vi "PH_Switch.destructor.vi"(0 "i ref in":refnum<vi>, 5 "error in(no error)":errorcluster) -> (19 "error out":errorcluster)   [LabVIEW 2014, in "PH_Switch.lvlib"]
doc: "This is the destructor of a class.\n\nLicense Agreement for this software:\n\nCopyright (C)\nGesellschaft für Schwerionenforschung, GSI\nPlanckstr. 1\n64291 Darmstadt\nGermany\n\nContact: D.Beck@gsi.de \n\nThis program is free software; you can redistribute it and/or modify it under the terms of the \nGNU General Public License as published by the Free Software Foundation; either version 2 of \nthe license, or (at your option) any later version.\n\nThis program is distributed in the hope that it will be useful, but WITHOUT ANY WARRANTY; \nwithout even the implied warranty of MERCHANTABILITY or FITNESS FOR A PARTICULAR PURPOSE. See the GNU General License for more details (http://www.gnu.org).\n\nGesellschaft für Schwerionenforschung, GSI\nPlanckstr. 1, 64291 Darmstadt, Germany\nFor all questions and ideas contact: M.Richter@gsi.de, H.Brand@gsi.de or D.Beck@gsi.de.\nLast update: 16-JUN-2004"
uses:
  PH_Switch.lvlib
  PH_PSDBWriter/PH_PSDBWriter.lvlib
  PH_StatusHandler/PH_StatusHandler.lvlib
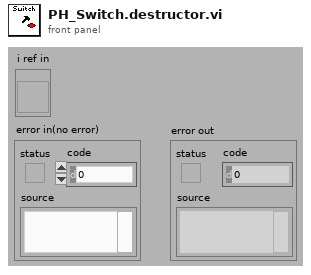
[diagram p1: front panel]
types:
  T1 = enum16{"SetAttribute", "GetAttribute", "CreateAttribute", "DestroyAttribute", "DestroyAllAtributes"}
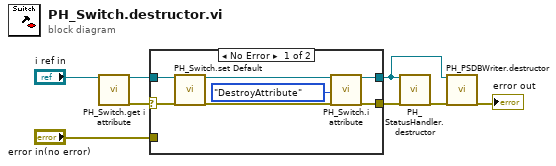
[diagram p0: block diagram]
diagram:
  n1 = call "PH_Switch.get i attribute.vi"("i ref in"="i ref in") -> ("i ref out"=w7:refnum<vi>, "error out"=w6:errorcluster)  [unwired: 16 in, 1 out]
  n2 = case shown="No Error" w6 {
    selector: w6 -> [w11 _]
    tunnel: [w14 w16] -> w1
    tunnel: [w13 w17] -> w4
    tunnel: w7 -> [w12 w16]
    tunnel: "error in(no error)" -> [_ w17]
    frame No Error {
      n3 = call "PH_Switch.set Default.vi"("i ref in"=w12, "error in"=w11) -> ("i ref out"=w10:refnum<vi>, "error out"=w9:errorcluster)  [unwired: 16 in]
      n4 = call "PH_Switch.i attribute.vi"("VI Refnum"=w10, "Action"=T1."DestroyAttribute", "error in (no error)"=w9) -> ("VI Refnum out"=w14:refnum<vi>, "error out"=w13:errorcluster)  [unwired: 14 in, 1 out]
    }
    frame Error {
    }
  }
  n5 = call "PH_StatusHandler.destructor.vi"("i ref in"=w1, "error in(no error)"=w4) -> ("error out"=w2:errorcluster)  [unwired: 17 in]
  n6 = call "PH_PSDBWriter.destructor.vi"("i ref in"=w1, "error in(no error)"=w2) -> ("error out"=→"error out":errorcluster)  [unwired: 17 in]
